vi "exercicio 2.vi"() -> ()   [LabVIEW 2025]
panel:
  in  "Boolean 3":bool
  out "s? t:f":dbl[](array[numeric])
  out "Boolean":bool
  out "String":string="opa"
  out "Slide":u8(slide) scale=0.0..200.0
  in  "Numeric":dbl
  in  "Array 2-1":dbl
  in  "Array 2-0":dbl
  in  "Array 1-0":dbl
  in  "Array 1-1":dbl
  out "i value":i32
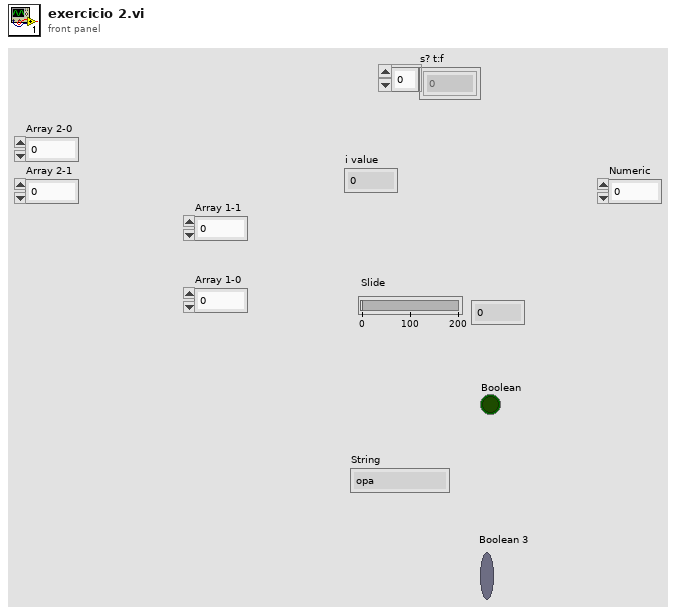
[diagram p1: front panel]
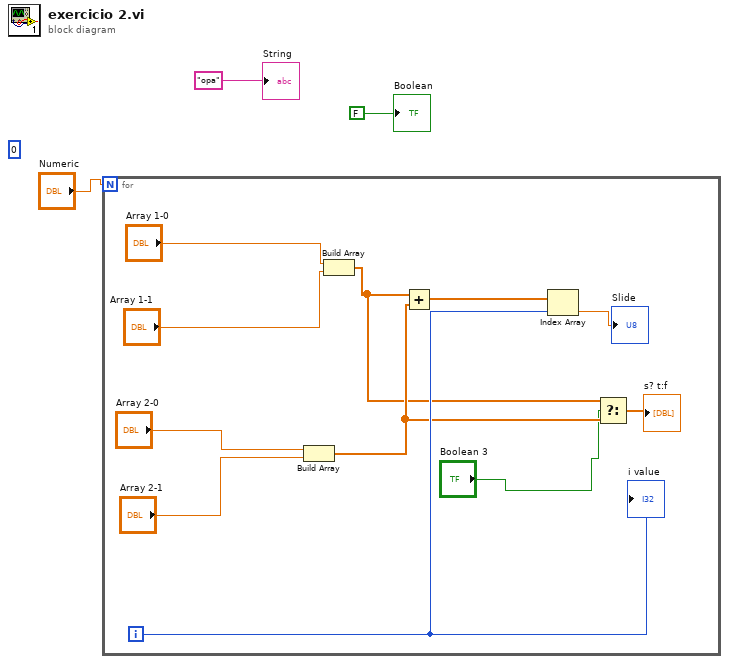
[diagram p0: block diagram]
diagram:
  (unwired) 0
  n1 = for {
    N: "Numeric" -> [_]
    i -> [w11]
    n2 = Build Array("Array 2-0", "Array 2-1") -> (w7:dbl[])
    n3 = Build Array("Array 1-0", "Array 1-1") -> (w6:dbl[])
    n4 = Add(x=w6, y=w7) -> (x+y=w8:dbl[])
    n5 = Index Array(array=w8, index=w11) -> (element=→"Slide":dbl)
    n6 = Select(t=w6, s="Boolean 3", f=w7) -> (s? t:f=→"s? t:f":dbl[])
    "i value" <- w11
  }
  "String" <- "opa"
  "Boolean" <- FALSE
